vi "SimpleProgram.vi"() -> ()   [LabVIEW 2018, in "LumencorDLL32.lvlib"]
uses:
  LumencorDLL32.lvlib
panel:
  out "lo(x)":u8
  out "hi(x)":u8
  out "Ready?":bool
  out "error out":errorcluster
  in  "error in (no error)":errorcluster
  in  "stop":bool
  in  "Intensity":dbl(slide) scale=0.0..100.0
  in  "On/Off":bool
  in  "VISA resource name":refnum<visa-resource-name>="COM3"
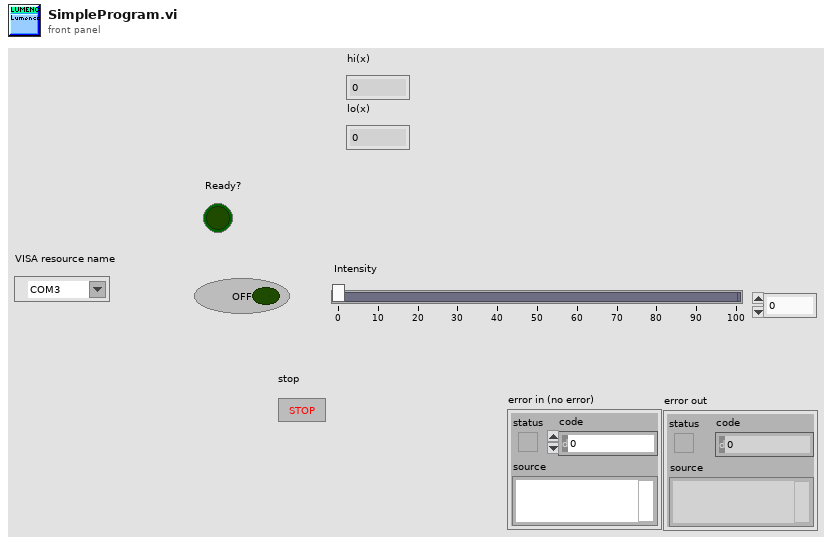
[diagram p1: front panel]
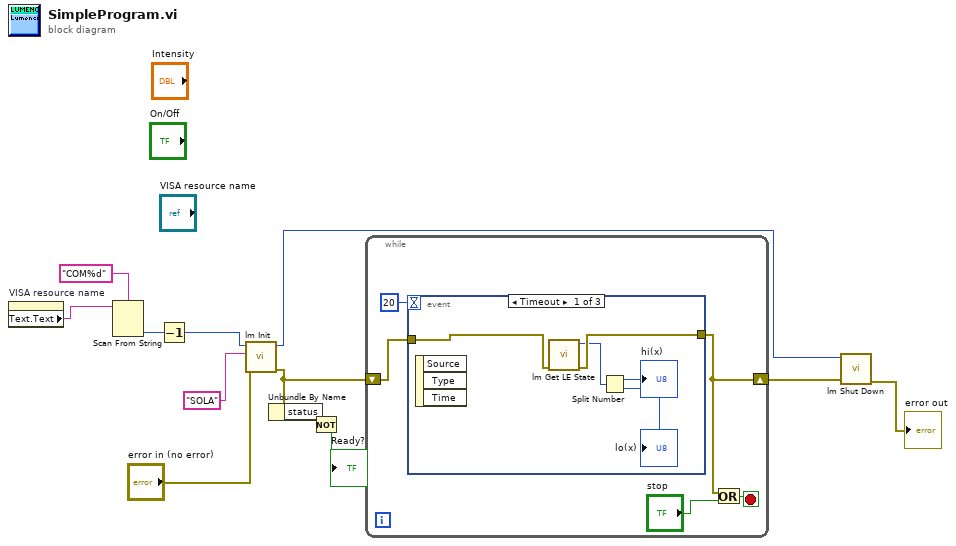
[diagram p0: block diagram]
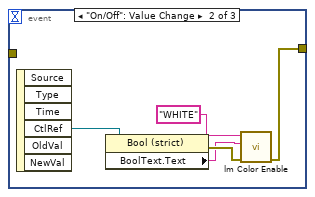
[diagram p2: hidden frame]
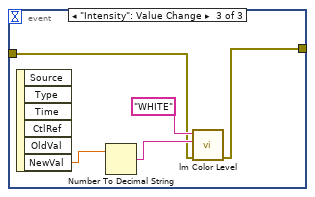
[diagram p3: hidden frame]
diagram:
  n1 = property on="VISA resource name" class="VISAName"() -> ("Text.Text"=w9:string)  [unwired: 2 in, 2 out]
  n2 = Scan From String(format string="COM%d", input string=w9) -> (output 1=w10:i32)  [unwired: 3 in, 3 out]
  n3 = Decrement(x=w10) -> (x-1=w8:i32)
  n4 = call "lm Init.vi"("error in (no error)"="error in (no error)", "LETypeStr"="SOLA", "ComPort"=w8) -> ("error out"=w3:errorcluster, "function return"=w2:u32)  [unwired: 6 in, 1 out]
  n5 = Unbundle By Name(w3) -> ("status"=w4:bool)
  n6 = Not(x=w4) -> (.not. x?=→"Ready?":bool)
  n7 = while {
    shift-right: [w15] -> w7
    shift-left: w3 -> [w17]
    stop <- w16 stop-if-true
    n8 = event shown="[0] Timeout" {
      selector: _ -> [_ _ _]
      dyn-events: _ -> [_ _ _]
      timeout: 20 -> [_ _ _]
      tunnel: w17 -> [w22 _ w29]
      tunnel: [w21 w23 w28] -> w15
      event Timeout {
        n9 = event-data() -> ()  [unwired: 1 in, 3 out]
        n10 = call "lm Get LE State.vi"("error in (no error)"=w22) -> ("error out"=w21:errorcluster, "function return"=w20:i16)  [unwired: 9 in]
        n11 = Split Number(x=w20) -> (hi(x)=→"hi(x)":u8, lo(x)=→"lo(x)":u8)
      }
      event "On/Off": Value Change {
        n12 = event-data() -> ("CtlRef"=w25:refnum<vi>)  [unwired: 1 in, 5 out]
        n13 = property class="Bool (strict)"(reference=w25) -> (error out=w26:errorcluster, "BoolText.Text"=w24:string)  [unwired: 1 in, 1 out]
        n14 = call "lm Color Enable.vi"("error in (no error)"=w26, "str_State"=w24, "str_Color"="WHITE") -> ("error out"=w23:errorcluster)  [unwired: 6 in, 2 out]
      }
      event "Intensity": Value Change {
        n15 = event-data() -> ("NewVal"=w32:dbl)  [unwired: 1 in, 5 out]
        n16 = Number To Decimal String(number=w32) -> (decimal integer string=w31:string)  [unwired: 1 in]
        n17 = call "lm Color Level.vi"("error in (no error)"=w29, "str_Level"=w31, "str_Color"="WHITE") -> ("error out"=w28:errorcluster)  [unwired: 6 in, 2 out]
      }
    }
    n18 = Or(x=w15, y="stop") -> (x .or. y?=w16:bool)
  }
  n19 = call "lm Shut Down.vi"("error in (no error)"=w7, "hSerial"=w2) -> ("error out"=→"error out":errorcluster)  [unwired: 8 in, 1 out]
